vi "map.vi"(7 "value":dbl, 8 "new low 2":dbl, 9 "new high 2":dbl, 10 "low":dbl, 11 "high":dbl) -> (2 "new value":dbl)   [LabVIEW 2014]
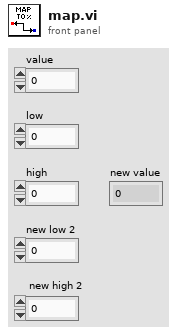
[diagram p1: front panel]
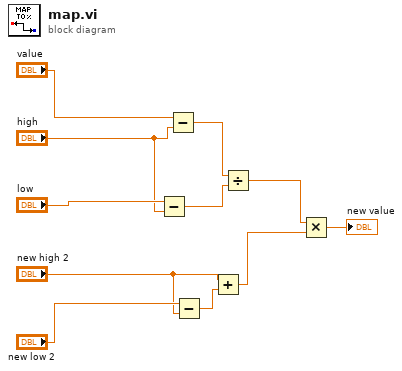
[diagram p0: block diagram]
diagram:
  n1 = Subtract(x="low", y="high") -> (x-y=w7:dbl)
  n2 = Subtract(x="value", y="high") -> (x-y=w10:dbl)
  n3 = Subtract(x="new low 2", y="new high 2") -> (x-y=w4:dbl)
  n4 = Add(x="new high 2", y=w4) -> (x+y=w2:dbl)
  n5 = Divide(x=w10, y=w7) -> (x/y=w6:dbl)
  n6 = Multiply(x=w6, y=w2) -> (x*y=→"new value":dbl)
